vi "Analog Replay Page.vi"(8 "error in (no error)":errorcluster, 11 "Node Ptr":T1 format="%.0x") -> (0 "error out":errorcluster)   [LabVIEW 2017, in "Engine Simulation Toolkit System Explorer.lvlib"]
uses:
  Engine Simulation Toolkit System Explorer.lvlib
  <vilib>/NI Veristand/Custom Device API/Custom Device Item Ref.ctl
  Position Reference.ctl
  <vilib>/NI Veristand/Custom Device API/Custom Device Channel Type.ctl
  Shared/Properties.vi
  <vilib>/NI Veristand/Custom Device API/Get Item Property (Double).vi
  <vilib>/NI Veristand/Custom Device API/Get Item Property (Boolean).vi
  <vilib>/NI Veristand/Custom Device API/Get Item Property (Dependent File).vi
  <vilib>/NI Veristand/Custom Device API/Get Item Property (U16).vi
  <vilib>/NI Veristand/Custom Device API/Get Item Property (String).vi
  <vilib>/NI Veristand/Custom Device API/Set Item Property (Double).vi
  <vilib>/NI Veristand/Custom Device API/Set Item Property (Boolean).vi
  Shared/Constants and GUIDs.vi
  <vilib>/NI Veristand/Custom Device Tools/Custom Device Utility Library/NI VeriStand - Search for Item by Name.vi
  <vilib>/NI Veristand/Custom Device API/Custom Device API.lvlib
  <vilib>/NI Veristand/Custom Device Tools/Custom Device Utility Library/Custom Device Utility Library.lvlib
  Shared/Engine Simulation Toolkit Shared.lvlib
panel:
  in  "Voltage below min speed":dbl=1.0 min=0.0 max=10.0
  out "Name in bitfile":string
  in  "Header":cluster{"Section Name":string}={"Section Name"="Analog Replay Settings"}
  in  "Name":string
  in  "DAC bipolar range (V)":dbl=0.0001 min=0.0001
  out "Data Graph":waveform(dbl)(graph)
  in  "Load":bool
  in  "VOverride":bool
  in  "ReverseNegate":bool
  out "Voltage XY":cluster{dbl, dbl}[](graph)
  in  "Voltage at max speed":dbl=1.0 min=0.0 max=10.0
  in  "Voltage at min speed":dbl=1.0 min=0.0 max=10.0
  in  "Min speed (RPM)":dbl=1.0 min=0.0
  in  "Max speed (RPM)":dbl=1.0 min=1.0
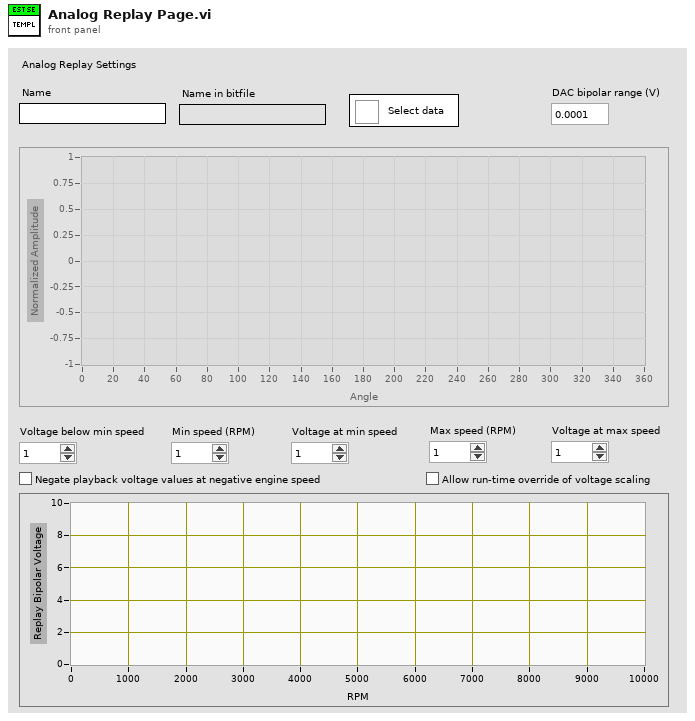
[diagram p1: front panel]
types:
  T1 = typedef "Custom Device API.lvlib/Custom Device Item Ref.ctl" = u64
  T2 = typedef "Custom Device API.lvlib/Custom Device Item Info.ctl" = cluster{"Name":string, "Is Channel":bool, "GUID":string, "Is Waveform":bool}
  T3 = enum8{"Enabled", "Disabled", "Disabled and Grayed Out"}
  T4 = typedef "Engine Simulation Toolkit System Explorer.lvlib/Position Reference.ctl" = enum16{"Crank angle", "Cycle angle"}
  T5 = typedef "Custom Device API.lvlib/Custom Device Channel Type.ctl" = enum16{"Input", "Output"}
  T6 = typedef "Custom Device API.lvlib/Custom Device Commands.ctl" = enum16{"Default", "Item renamed", "Shutdown", "Dynamic button pressed"}
  T7 = typedef "Engine Simulation Toolkit Shared.lvlib/Channel.ctl" = cluster{"Name":string, "Units":string, "Default":dbl, "Description":string, "Scalable":bool}
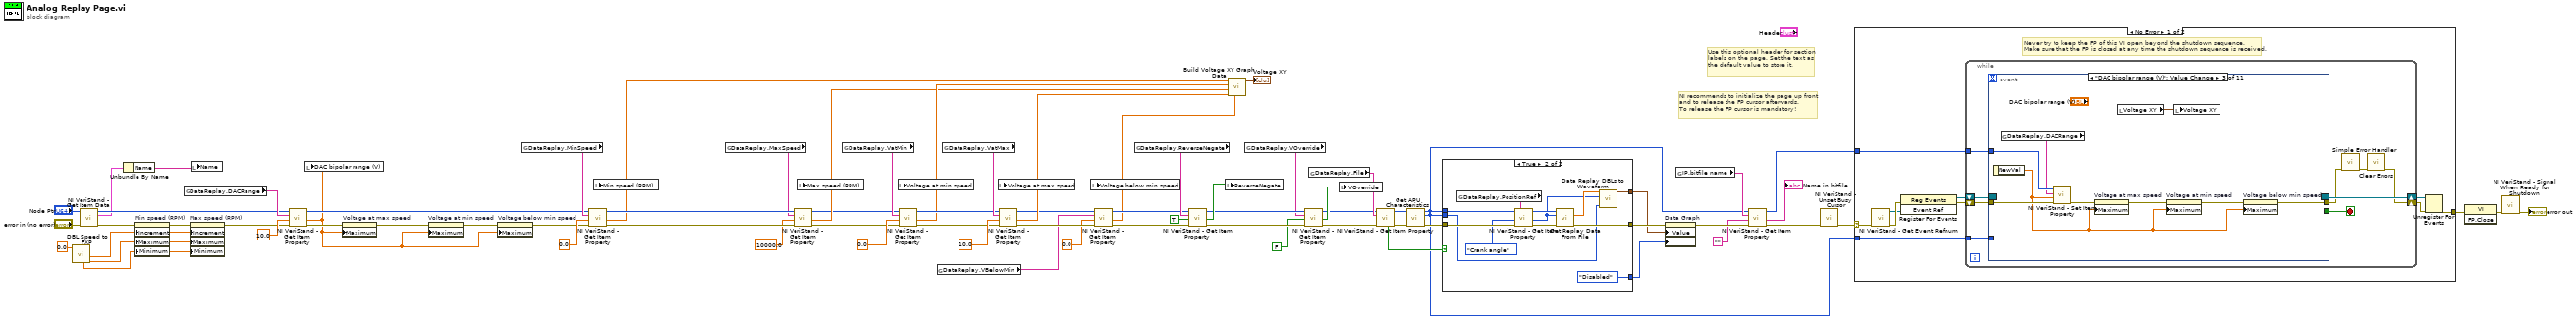
[diagram p0: block diagram]
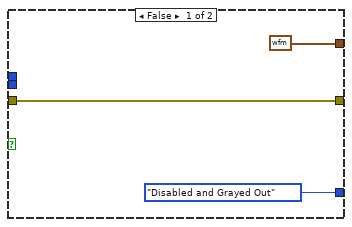
[diagram p2: hidden frame]
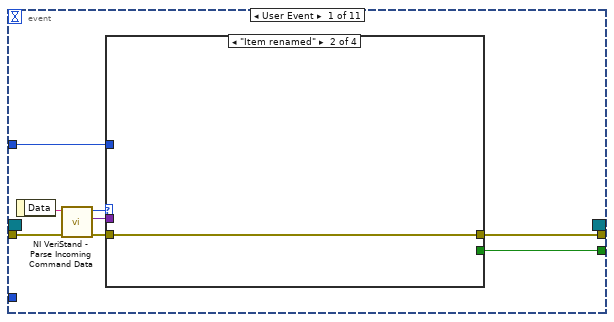
[diagram p3: hidden frame]
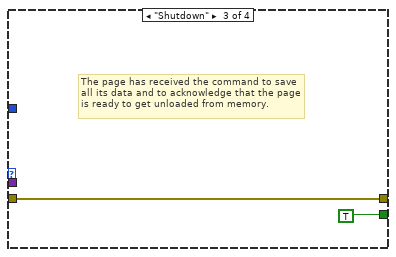
[diagram p5: hidden frame]
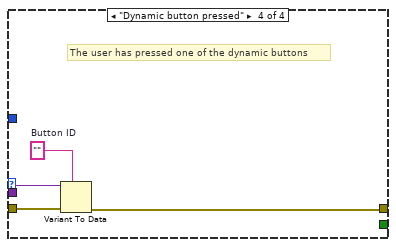
[diagram p6: hidden frame]
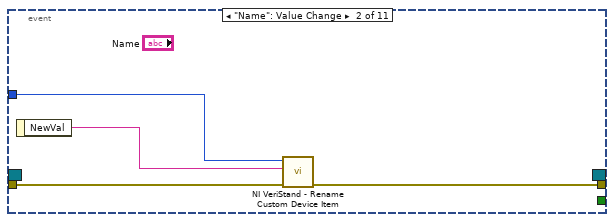
[diagram p7: hidden frame]
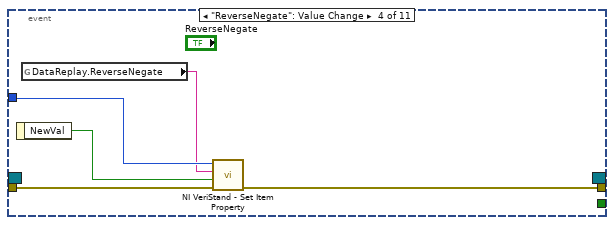
[diagram p8: hidden frame]
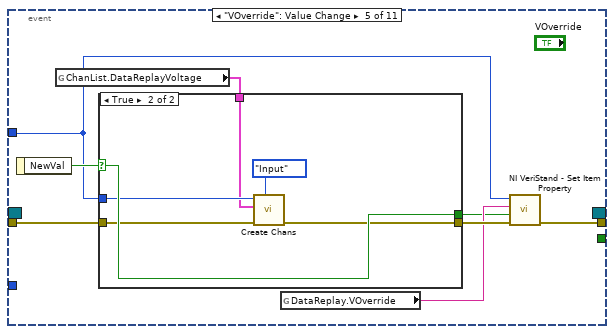
[diagram p9: hidden frame]
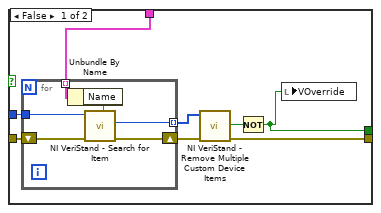
[diagram p10: hidden frame]
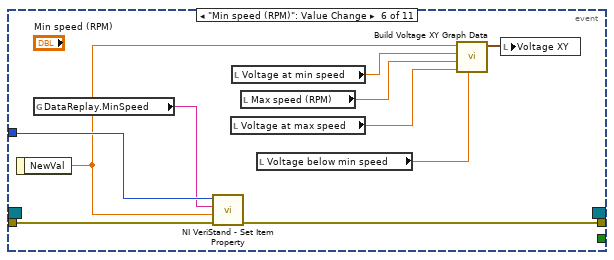
[diagram p11: hidden frame]
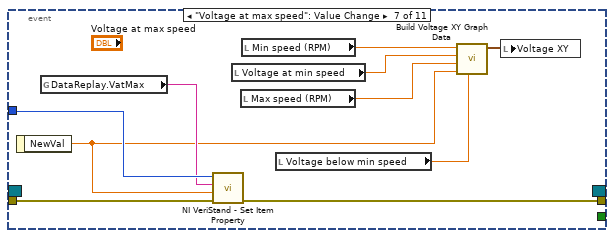
[diagram p12: hidden frame]
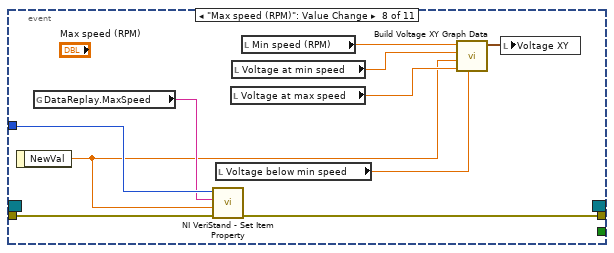
[diagram p13: hidden frame]
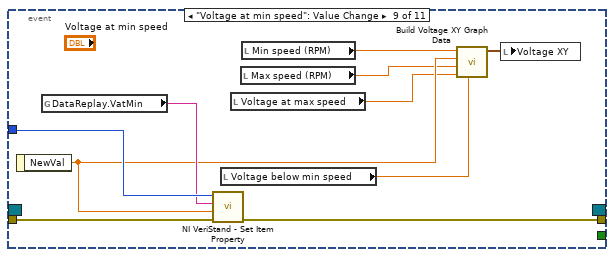
[diagram p14: hidden frame]
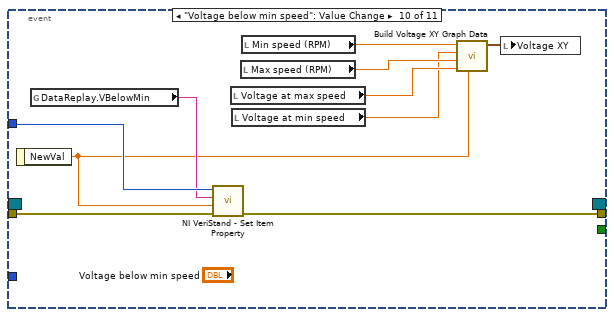
[diagram p15: hidden frame]
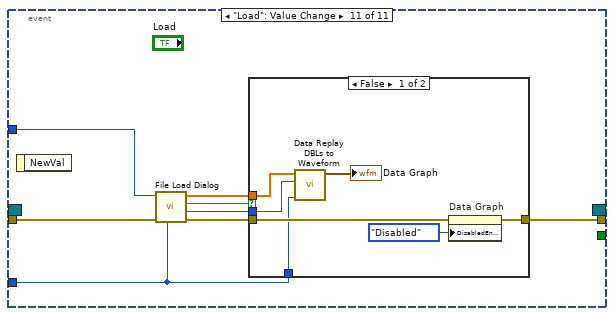
[diagram p16: hidden frame]
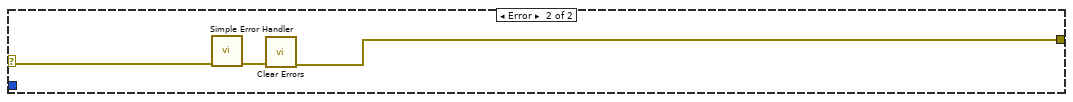
[diagram p18: hidden frame]
diagram:
  # "Use this optional header for section labels on the page. Set the text as the default value to store it."
  # "NI recommends to initialize the page up front\nand to release the FP cursor afterwards.\nTo release the FP cursor is mandatory!"
  n1 = call "DBL Speed to FXP.vi"("Desired speed (RPM)"=0.0) -> ("rpm max"=w3:dbl, "rpm resolution"=w4:dbl, "rpm min"=w2:dbl)  [unwired: 6 in, 2 out]
  n2 = call <vilib>:"NI VeriStand - Get Item Data.vi"("error in (no error)"="error in (no error)", "Item Ref in"="Node Ptr") -> ("error out"=w6:errorcluster, "Item Info"=w13:T2, "Item Ref out"=w14:T1)  [unwired: 6 in, 1 out]
  n3 = Unbundle By Name(w13) -> ("Name"=w12:string)
  n4 = property on="Min speed (RPM)" class="DigNum (strict)"(error in=w6, "Increment"=w4, "Maximum"=w3, "Minimum"=w2) -> (error out=w7:errorcluster)  [unwired: 1 in, 1 out]
  n5 = global read "Properties.vi" "DataReplay.DACRange"() -> (w28:string)
  n6 = property on="Max speed (RPM)" class="DigNum (strict)"(error in=w7, "Increment"=w4, "Maximum"=w3, "Minimum"=w2) -> (error out=w5:errorcluster)  [unwired: 1 in, 1 out]
  n7 = local write "Name"(w12) -> ()
  n8 = call-poly <vilib>:"NI VeriStand - Get Item Property.vi"("error in (no error)"=w5, "Default Value"=10.0, "Property Name"=w28, "Item Ref in"=w14) -> ("error out"=w26:errorcluster, "Value"=w18:dbl, "Item Ref out"=w29:T1)  [unwired: 4 in, 1 out]
  n9 = local write "DAC bipolar range (V)"(w18) -> ()
  n10 = property on="Voltage at max speed" class="DigNum (strict)"(error in=w26, "Maximum"=w18) -> (error out=w25:errorcluster)  [unwired: 1 in, 1 out]
  n11 = property on="Voltage at min speed" class="DigNum (strict)"(error in=w25, "Maximum"=w18) -> (error out=w19:errorcluster)  [unwired: 1 in, 1 out]
  n12 = property on="Voltage below min speed" class="DigNum (strict)"(error in=w19, "Maximum"=w18) -> (error out=w17:errorcluster)  [unwired: 1 in, 1 out]
  n13 = global read "Properties.vi" "DataReplay.MinSpeed"() -> (w71:string)
  n14 = call-poly <vilib>:"NI VeriStand - Get Item Property.vi"("error in (no error)"=w17, "Default Value"=0.0, "Property Name"=w71, "Item Ref in"=w29) -> ("error out"=w70:errorcluster, "Value"=w59:dbl, "Item Ref out"=w69:T1)  [unwired: 4 in, 1 out]
  n15 = local write "Min speed (RPM)"(w59) -> ()
  n16 = global read "Properties.vi" "DataReplay.MaxSpeed"() -> (w67:string)
  n17 = call-poly <vilib>:"NI VeriStand - Get Item Property.vi"("error in (no error)"=w70, "Default Value"=10000.0, "Property Name"=w67, "Item Ref in"=w69) -> ("error out"=w53:errorcluster, "Value"=w56:dbl, "Item Ref out"=w54:T1)  [unwired: 4 in, 1 out]
  n18 = local write "Max speed (RPM)"(w56) -> ()
  n19 = global read "Properties.vi" "DataReplay.VatMin"() -> (w65:string)
  n20 = call-poly <vilib>:"NI VeriStand - Get Item Property.vi"("error in (no error)"=w53, "Default Value"=0.0, "Property Name"=w65, "Item Ref in"=w54) -> ("error out"=w61:errorcluster, "Value"=w57:dbl, "Item Ref out"=w62:T1)  [unwired: 4 in, 1 out]
  n21 = local write "Voltage at min speed"(w57) -> ()
  n22 = global read "Properties.vi" "DataReplay.VBelowMin"() -> (w21:string)
  n23 = global read "Properties.vi" "DataReplay.VatMax"() -> (w64:string)
  n24 = call-poly <vilib>:"NI VeriStand - Get Item Property.vi"("error in (no error)"=w61, "Default Value"=10.0, "Property Name"=w64, "Item Ref in"=w62) -> ("error out"=w60:errorcluster, "Value"=w55:dbl, "Item Ref out"=w23:T1)  [unwired: 4 in, 1 out]
  n25 = local write "Voltage at max speed"(w55) -> ()
  n26 = call-poly <vilib>:"NI VeriStand - Get Item Property.vi"("error in (no error)"=w60, "Default Value"=0.0, "Property Name"=w21, "Item Ref in"=w23) -> ("error out"=w24:errorcluster, "Value"=w16:dbl, "Item Ref out"=w22:T1)  [unwired: 4 in, 1 out]
  n27 = local write "Voltage below min speed"(w16) -> ()
  n28 = global read "Properties.vi" "DataReplay.ReverseNegate"() -> (w51:string)
  n29 = call-poly <vilib>:"NI VeriStand - Get Item Property.vi"("error in (no error)"=w24, "Default Value"=TRUE, "Property Name"=w51, "Item Ref in"=w22) -> ("error out"=w52:errorcluster, "Value"=w50:bool, "Item Ref out"=w48:T1)  [unwired: 4 in, 1 out]
  n30 = local write "ReverseNegate"(w50) -> ()
  n31 = call "Build Voltage XY Graph Data.vi"("voltage below min"=w16, "maximum voltage"=w55, "maximum speed"=w56, "min voltage"=w57, "min speed"=w59) -> ("XY data"=→"Voltage XY":cluster{dbl, dbl}[])  [unwired: 6 in]
  n32 = global read "Properties.vi" "DataReplay.VOverride"() -> (w47:string)
  n33 = call-poly <vilib>:"NI VeriStand - Get Item Property.vi"("error in (no error)"=w52, "Default Value"=FALSE, "Property Name"=w47, "Item Ref in"=w48) -> ("error out"=w30:errorcluster, "Value"=w46:bool, "Item Ref out"=w31:T1)  [unwired: 4 in, 1 out]
  n34 = global read "Properties.vi" "DataReplay.File"() -> (w44:string)
  n35 = local write "VOverride"(w46) -> ()
  n36 = call-poly <vilib>:"NI VeriStand - Get Item Property.vi"("error in (no error)"=w30, "Property Name"=w44, "Item Ref in"=w31) -> ("error out"=w42:errorcluster, "Item Ref out"=w10:T1, "Found"=w43:bool)  [unwired: 4 in, 2 out]
  n37 = call "Get APU Characteristics.vi"("error in (no error)"=w42, "Item Ref in"=w10) -> ("error out"=w11:errorcluster, "total angle span (degrees)"=w8:u16, "Item Ref out"=w9:T1)  [unwired: 3 in, 4 out]
  n38 = case shown="True" w43 {
    tunnel: w9 -> [_ w87]
    tunnel: w11 -> [w79 w86]
    tunnel: [w79 w85] -> w40
    tunnel: [T3."Disabled and Grayed Out" ("Disabled") T3."Disabled" ("Disabled")] -> w41
    tunnel: [waveform(dbl) {"t0"=timestamp(0 s since 1904-01-01), "dt"=1.0, "Y"=[]} ("Data Graph") w90] -> w39
    tunnel: w8 -> [_ w84]
    frame False {
    }
    frame True {
      n39 = global read "Properties.vi" "DataReplay.PositionRef"() -> (w88:string)
      n40 = call-poly <vilib>:"NI VeriStand - Get Item Property.vi"("error in (no error)"=w86, "Default Value"=Position_Reference."Crank angle" ("Position reference"), "Property Name"=w88, "Item Ref in"=w87) -> ("error out"=w82:errorcluster, "Value"=w80:u16, "Item Ref out"=w81:T1)  [unwired: 4 in, 1 out]
      n41 = call "Get Replay Data From File.vi"("error in (no error)"=w82, "Position reference"=w80, "Item Ref in"=w81) -> ("error out"=w85:errorcluster, "DBL Data"=w91:dbl[])  [unwired: 6 in, 1 out]
      n42 = call "Data Replay DBLs to Waveform.vi"("cycle range"=w84, "Position reference"=w80, "Data"=w91) -> ("waveform"=w90:waveform(dbl))  [unwired: 8 in]
    }
  }
  n43 = property on="Data Graph" class="WFGraph (strict)"(error in=w40, "Value"=w39, "DisabledEnum"=w41) -> (error out=w38:errorcluster)  [unwired: 1 in, 1 out]
  n44 = global read "Properties.vi" "IP.bitfile name"() -> (w35:string)
  n45 = call-poly <vilib>:"NI VeriStand - Get Item Property.vi"("error in (no error)"=w38, "Default Value"="", "Property Name"=w35, "Item Ref in"=w9) -> ("error out"=w37:errorcluster, "Value"=→"Name in bitfile":string, "Item Ref out"=w36:T1)  [unwired: 4 in, 1 out]
  n46 = call <vilib>:"NI VeriStand - Unset Busy Cursor.vi"("error in (no error)"=w37) -> ("error out"=w73:errorcluster)  [unwired: 10 out]
  n47 = case shown="No Error" w73 {
    selector: w73 -> [w93 w241]
    tunnel: [w98 w239] -> w76
    tunnel: w36 -> [w94 _]
    tunnel: w8 -> [w92 _]
    frame No Error {
      # "Never try to keep the FP of this VI open beyond the shutdown sequence.\nMake sure that the FP is closed at any time the shutdown sequence is received."
      n48 = call <vilib>:"NI VeriStand - Get Event Refnum.vi"("error in (no error)"=w93) -> ("error out"=w101:errorcluster, "Event Ref"=w97:refnum<user-event>)  [unwired: 9 out]
      n49 = register-events(error in=w101, w97) -> (reference out=w95:refnum<event-registration>, error out=w96:errorcluster)  [unwired: 1 in]
      n50 = while {
        tunnel: w94 -> [w106]
        shift-right: [w103] -> w99
        shift-left: w96 -> [w109]
        shift-right: [w110] -> w100
        shift-left: w95 -> [w108]
        tunnel: w92 -> [w102]
        stop <- w107 stop-if-true
        n51 = event shown="[2] \"DAC bipolar range (V)\": Value Change" {
          selector: w108 -> [_ _ _ _ _ _ _ _ _ _ _]
          dyn-events: [_ _ _ _ _ _ _ _ _ _ _] -> w110
          timeout: _ -> [_ _ _ _ _ _ _ _ _ _ _]
          tunnel: w109 -> [w118 w130 w139 w144 w150 w182 w192 w202 w212 w222 w230]
          tunnel: [w114 _ _ _ _ _ _ _ _ _ _] -> w107
          tunnel: [w113 w129 w133 w140 w148 w179 w189 w199 w209 w219 w229] -> w105
          tunnel: w106 -> [w112 w128 w138 w143 w147 w181 w191 w201 w211 w221 w226]
          tunnel: w102 -> [_ _ _ _ _ _ _ _ _ _ w223]
          event User Event {
            n52 = event-data() -> ("Data"=w117:string)  [unwired: 1 out]
            n53 = call <vilib>:"NI VeriStand - Parse Incoming Command Data.vi"("error in (no error)"=w118, "Incoming data"=w117) -> ("error out"=w116:errorcluster, "Outgoing data"=w111:variant, "Action"=w115:T6)  [unwired: 7 out]
            n54 = case shown="\"Item renamed\"" w115 {
              tunnel: w116 -> [w119 w120 w121 w126]
              tunnel: [_ _ TRUE _] -> w114
              tunnel: [w119 w120 w121 w123] -> w113
              tunnel: w112 -> [_ _ _ _]
              tunnel: w111 -> [_ _ _ w125]
              frame "Default", Default {
              }
              frame "Item renamed" {
              }
              frame "Shutdown" {
                # "The page has received the command to save all its data and to acknowledge that the page is ready to get unloaded from memory."
              }
              frame "Dynamic button pressed" {
                w124 = ""  # Button ID
                # "The user has pressed one of the dynamic buttons"
                n55 = Variant To Data(error in=w126, type=w124, Variant=w125) -> (error out=w123:errorcluster)  [unwired: 1 out]
              }
            }
          }
          event "Name": Value Change {
            n56 = event-data() -> ("NewVal"=w127:string)  [unwired: 1 out]
            n57 = call <vilib>:"NI VeriStand - Rename Custom Device Item.vi"("error in (no error)"=w130, "New Name"=w127, "Item Ref in"=w128) -> ("error out"=w129:errorcluster)  [unwired: 1 in, 7 out]
          }
          event "DAC bipolar range (V)": Value Change {
            n58 = event-data() -> ("NewVal"=w132:dbl)  [unwired: 1 out]
            n59 = global read "Properties.vi" "DataReplay.DACRange"() -> (w137:string)
            n60 = call-poly <vilib>:"NI VeriStand - Set Item Property.vi"("error in (no error)"=w139, "Value"=w132, "Property Name"=w137, "Item Ref in"=w138) -> ("error out"=w136:errorcluster)  [unwired: 5 in, 2 out]
            n61 = property on="Voltage at max speed" class="DigNum (strict)"(error in=w136, "Maximum"=w132) -> (error out=w135:errorcluster)  [unwired: 1 in, 1 out]
            n62 = local read "Voltage XY"() -> (w131:cluster{dbl, dbl}[])
            n63 = property on="Voltage at min speed" class="DigNum (strict)"(error in=w135, "Maximum"=w132) -> (error out=w134:errorcluster)  [unwired: 1 in, 1 out]
            n64 = local write "Voltage XY"(w131) -> ()
            n65 = property on="Voltage below min speed" class="DigNum (strict)"(error in=w134, "Maximum"=w132) -> (error out=w133:errorcluster)  [unwired: 1 in, 1 out]
          }
          event "ReverseNegate": Value Change {
            n66 = event-data() -> ("NewVal"=w142:bool)  [unwired: 1 out]
            n67 = global read "Properties.vi" "DataReplay.ReverseNegate"() -> (w141:string)
            n68 = call-poly <vilib>:"NI VeriStand - Set Item Property.vi"("error in (no error)"=w144, "Value"=w142, "Property Name"=w141, "Item Ref in"=w143) -> ("error out"=w140:errorcluster)  [unwired: 5 in, 2 out]
          }
          event "VOverride": Value Change {
            n69 = event-data() -> ("NewVal"=w152:bool)  [unwired: 1 out]
            n70 = global read "Constants and GUIDs.vi" "ChanList.DataReplayVoltage"() -> (w151:T7[])
            n71 = case shown="True" w152 {
              selector: w152 -> [_ w172]
              tunnel: w150 -> [w160 w171]
              tunnel: w147 -> [w159 w169]
              tunnel: w151 -> [w158 w168]
              tunnel: [w154 w170] -> w149
              tunnel: [w153 w172] -> w145
              frame False {
                n72 = for {
                  tunnel: w159 -> [w165]
                  tunnel: w158 -> [w162] mode=indexing
                  shift-right: [w164] -> w157
                  shift-left: w160 -> [w166]
                  tunnel: [w163] -> w156 mode=indexing
                  n73 = Unbundle By Name(w162) -> ("Name"=w161:string)
                  n74 = call-poly <vilib>:"NI VeriStand - Search for Item.vi"("error in"=w166, "Item Name"=w161, "Section Ref in"=w165) -> ("error out"=w164:errorcluster, "Item Ref"=w163:T1)  [unwired: 5 in, 2 out]
                }
                n75 = call <vilib>:"NI VeriStand - Remove Multiple Custom Device Items.vi"("error in (no error)"=w157, "Item Refs in"=w156) -> ("error out"=w154:errorcluster, "Deleted?"=w155:bool)  [unwired: 8 in]
                n76 = Not(x=w155) -> (.not. x?=w153:bool)
                n77 = local write "VOverride"(w153) -> ()
              }
              frame True {
                n78 = call "Create Chans.vi"("Type"=Custom_Device_Channel_Type."Input", "error in (no error)"=w171, "Channels"=w168, "Section Ptr"=w169) -> ("error out"=w170:errorcluster)  [unwired: 4 in, 3 out]
              }
            }
            n79 = global read "Properties.vi" "DataReplay.VOverride"() -> (w146:string)
            n80 = call-poly <vilib>:"NI VeriStand - Set Item Property.vi"("error in (no error)"=w149, "Value"=w145, "Property Name"=w146, "Item Ref in"=w147) -> ("error out"=w148:errorcluster)  [unwired: 5 in, 2 out]
          }
          event "Min speed (RPM)": Value Change {
            n81 = event-data() -> ("NewVal"=w174:dbl)  [unwired: 1 out]
            n82 = global read "Properties.vi" "DataReplay.MinSpeed"() -> (w180:string)
            n83 = call-poly <vilib>:"NI VeriStand - Set Item Property.vi"("error in (no error)"=w182, "Value"=w174, "Property Name"=w180, "Item Ref in"=w181) -> ("error out"=w179:errorcluster)  [unwired: 5 in, 2 out]
            n84 = local read "Voltage at max speed"() -> (w177:dbl)
            n85 = local read "Voltage at min speed"() -> (w175:dbl)
            n86 = local read "Max speed (RPM)"() -> (w176:dbl)
            n87 = local read "Voltage below min speed"() -> (w173:dbl)
            n88 = call "Build Voltage XY Graph Data.vi"("voltage below min"=w173, "maximum voltage"=w177, "maximum speed"=w176, "min voltage"=w175, "min speed"=w174) -> ("XY data"=w178:cluster{dbl, dbl}[])  [unwired: 6 in]
            n89 = local write "Voltage XY"(w178) -> ()
          }
          event "Voltage at max speed": Value Change {
            n90 = event-data() -> ("NewVal"=w184:dbl)  [unwired: 1 out]
            n91 = global read "Properties.vi" "DataReplay.VatMax"() -> (w190:string)
            n92 = call-poly <vilib>:"NI VeriStand - Set Item Property.vi"("error in (no error)"=w192, "Value"=w184, "Property Name"=w190, "Item Ref in"=w191) -> ("error out"=w189:errorcluster)  [unwired: 5 in, 2 out]
            n93 = local read "Voltage at min speed"() -> (w186:dbl)
            n94 = local read "Max speed (RPM)"() -> (w185:dbl)
            n95 = local read "Min speed (RPM)"() -> (w187:dbl)
            n96 = local read "Voltage below min speed"() -> (w183:dbl)
            n97 = call "Build Voltage XY Graph Data.vi"("voltage below min"=w183, "maximum voltage"=w184, "maximum speed"=w185, "min voltage"=w186, "min speed"=w187) -> ("XY data"=w188:cluster{dbl, dbl}[])  [unwired: 6 in]
            n98 = local write "Voltage XY"(w188) -> ()
          }
          event "Max speed (RPM)": Value Change {
            n99 = event-data() -> ("NewVal"=w194:dbl)  [unwired: 1 out]
            n100 = global read "Properties.vi" "DataReplay.MaxSpeed"() -> (w200:string)
            n101 = call-poly <vilib>:"NI VeriStand - Set Item Property.vi"("error in (no error)"=w202, "Value"=w194, "Property Name"=w200, "Item Ref in"=w201) -> ("error out"=w199:errorcluster)  [unwired: 5 in, 2 out]
            n102 = local read "Voltage below min speed"() -> (w193:dbl)
            n103 = local read "Voltage at max speed"() -> (w196:dbl)
            n104 = local read "Voltage at min speed"() -> (w195:dbl)
            n105 = local read "Min speed (RPM)"() -> (w197:dbl)
            n106 = call "Build Voltage XY Graph Data.vi"("voltage below min"=w193, "maximum voltage"=w196, "maximum speed"=w194, "min voltage"=w195, "min speed"=w197) -> ("XY data"=w198:cluster{dbl, dbl}[])  [unwired: 6 in]
            n107 = local write "Voltage XY"(w198) -> ()
          }
          event "Voltage at min speed": Value Change {
            n108 = event-data() -> ("NewVal"=w206:dbl)  [unwired: 1 out]
            n109 = global read "Properties.vi" "DataReplay.VatMin"() -> (w210:string)
            n110 = call-poly <vilib>:"NI VeriStand - Set Item Property.vi"("error in (no error)"=w212, "Value"=w206, "Property Name"=w210, "Item Ref in"=w211) -> ("error out"=w209:errorcluster)  [unwired: 5 in, 2 out]
            n111 = local read "Voltage below min speed"() -> (w203:dbl)
            n112 = local read "Voltage at max speed"() -> (w205:dbl)
            n113 = local read "Max speed (RPM)"() -> (w204:dbl)
            n114 = local read "Min speed (RPM)"() -> (w207:dbl)
            n115 = call "Build Voltage XY Graph Data.vi"("voltage below min"=w203, "maximum voltage"=w205, "maximum speed"=w204, "min voltage"=w206, "min speed"=w207) -> ("XY data"=w208:cluster{dbl, dbl}[])  [unwired: 6 in]
            n116 = local write "Voltage XY"(w208) -> ()
          }
          event "Voltage below min speed": Value Change {
            n117 = event-data() -> ("NewVal"=w213:dbl)  [unwired: 1 out]
            n118 = global read "Properties.vi" "DataReplay.VBelowMin"() -> (w220:string)
            n119 = call-poly <vilib>:"NI VeriStand - Set Item Property.vi"("error in (no error)"=w222, "Value"=w213, "Property Name"=w220, "Item Ref in"=w221) -> ("error out"=w219:errorcluster)  [unwired: 5 in, 2 out]
            n120 = local read "Voltage at max speed"() -> (w216:dbl)
            n121 = local read "Voltage at min speed"() -> (w214:dbl)
            n122 = local read "Max speed (RPM)"() -> (w215:dbl)
            n123 = local read "Min speed (RPM)"() -> (w217:dbl)
            n124 = call "Build Voltage XY Graph Data.vi"("voltage below min"=w213, "maximum voltage"=w216, "maximum speed"=w215, "min voltage"=w214, "min speed"=w217) -> ("XY data"=w218:cluster{dbl, dbl}[])  [unwired: 6 in]
            n125 = local write "Voltage XY"(w218) -> ()
          }
          event "Load": Value Change {
            n126 = event-data() -> ()  [unwired: 2 out]
            n127 = call "File Load Dialog.vi"("cycle range"=w223, "error in (no error)"=w230, "Node Ptr"=w226) -> ("error out"=w228:errorcluster, "Position reference"=w224:T4, "Cancelled"=w227:bool, "Data"=w225:dbl[])  [unwired: 5 in]
            n128 = case shown="False" w227 {
              tunnel: [w236 w238] -> w229
              tunnel: w228 -> [w237 w238]
              tunnel: w225 -> [w234 _]
              tunnel: w224 -> [w232 _]
              tunnel: w223 -> [w231 _]
              frame False {
                n129 = call "Data Replay DBLs to Waveform.vi"("cycle range"=w231, "Position reference"=w232, "Data"=w234) -> ("waveform"=→"Data Graph":waveform(dbl))  [unwired: 8 in]
                n130 = property on="Data Graph" class="WFGraph (strict)"(error in=w237, "DisabledEnum"=T3."Disabled" ("Disabled")) -> (error out=w236:errorcluster)  [unwired: 1 in, 1 out]
              }
              frame True {
              }
            }
          }
        }
        n131 = call <vilib>:"Simple Error Handler.vi"("error in (no error)"=w105) -> ("error out"=w104:errorcluster)  [unwired: 1 in, 7 out]
        n132 = call <vilib>:"Clear Errors.vi"("error in (no error)"=w104) -> ("error out"=w103:errorcluster)  [unwired: 1 in, 5 out]
      }
      n133 = Unregister For Events(event registration refnum=w100, error in=w99) -> (error out=w98:errorcluster)
    }
    frame Error {
      n134 = call <vilib>:"Simple Error Handler.vi"("error in (no error)"=w241) -> ("error out"=w240:errorcluster)  [unwired: 1 in, 7 out]
      n135 = call <vilib>:"Clear Errors.vi"("error in (no error)"=w240) -> ("error out"=w239:errorcluster)  [unwired: 1 in, 5 out]
    }
  }
  n136 = invoke class="VI" method="FP.Close"(error in=w76) -> (error out=w75:errorcluster)  [unwired: 2 in, 2 out]
  n137 = call <vilib>:"NI VeriStand - Signal When Ready for Shutdown.vi"("error in (no error)"=w75) -> ("error out"=→"error out":errorcluster)  [unwired: 10 out]
